vi "SetRcvrAttn.vi"(0 "VISA IN":refnum<visa-resource-name>="PNA", 5 "error in":errorcluster) -> (14 "VISA Out":refnum<visa-resource-name>, 19 "error out":errorcluster)   [LabVIEW 2018, in "PNA-X.lvlib"]
uses:
  PNA-X.lvlib
panel:
  in  "RxType":string(combo)
  in  "Attenuation":string(combo)
  in  "Channel":i32=1
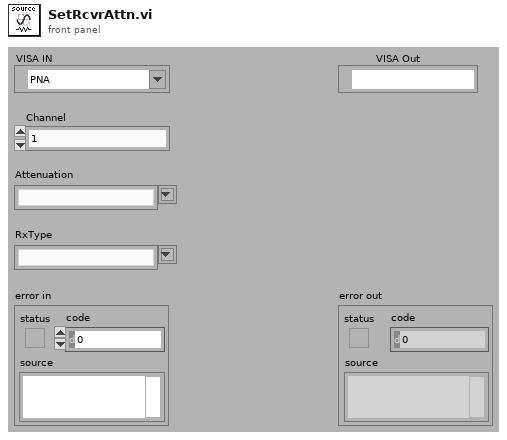
[diagram p1: front panel]
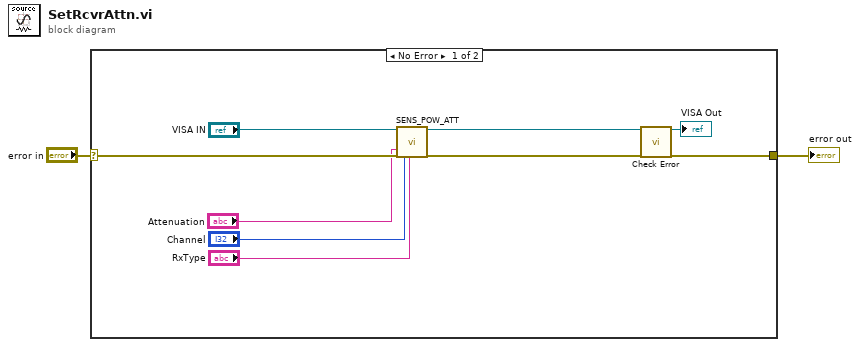
[diagram p0: block diagram]
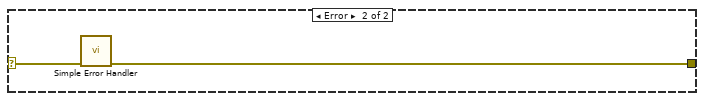
[diagram p2: hidden frame]
diagram:
  n1 = case shown="No Error" "error in" {
    selector: "error in" -> [w9 w13]
    tunnel: [w11 w12] -> w2
    frame No Error {
      n2 = call "SENS_POW_ATT.vi"("VISA IN"="VISA IN", "Attenuation"="Attenuation", "error in"=w9, "Channel"="Channel", "RxType"="RxType") -> ("VISA Out"=w5:refnum<visa-resource-name>, "error out"=w8:errorcluster)  [unwired: 13 in]
      n3 = call "Check Error.vi"("VISA Resource Name"=w5, "error in (no error)"=w8) -> ("dup VISA session"=→"VISA Out":refnum<visa-resource-name>, "error out"=w11:errorcluster)  [unwired: 16 in]
    }
    frame Error {
      n4 = call <vilib>:"Simple Error Handler.vi"("error in (no error)"=w13) -> ("error out"=w12:errorcluster)  [unwired: 4 in, 4 out]
    }
  }
  "error out" <- w2
